vi "Stack_Sequence.vi"() -> ()   [LabVIEW 2016]
panel:
  out "x+y":dbl
  out "Triangle":dynamicdata(graph)
  out "Sine":dynamicdata(graph)
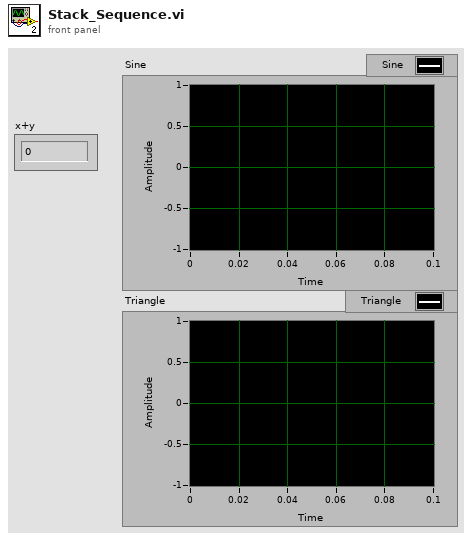
[diagram p1: front panel]
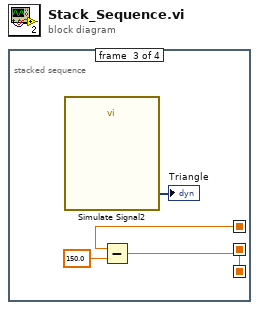
[diagram p0: block diagram]
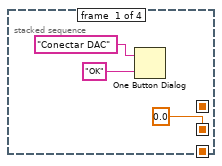
[diagram p2: hidden frame]
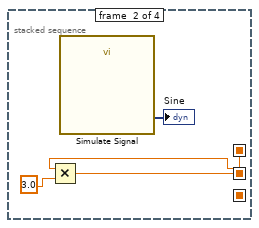
[diagram p3: hidden frame]
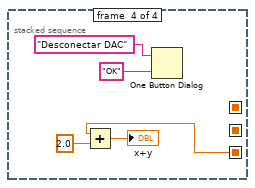
[diagram p4: hidden frame]
diagram:
  n1 = stacked-sequence {
    seq-local: [0.0 _ _ _] -> [_ w5 _ _]
    seq-local: [_ w4 _ _] -> [_ _ w9 _]
    seq-local: [_ _ w8 _] -> [_ _ _ w14]
    frame #0 {
      n2 = One Button Dialog(message="Conectar DAC", button name ("OK")="OK") -> ()  [unwired: 1 out]
    }
    frame #1 {
      n3 = Multiply(x=w5, y=3.0) -> (x*y=w4:dbl)
      n4 = call "Simulate Signal"() -> ("Sine"=→"Sine":dynamicdata)  [unwired: 14 in, 1 out]
    }
    frame #2 {
      n5 = call "Simulate Signal2"() -> ("Triangle"=→"Triangle":dynamicdata)  [unwired: 14 in, 1 out]
      n6 = Subtract(x=w9, y=150.0) -> (x-y=w8:dbl)
    }
    frame #3 {
      n7 = Add(x=w14, y=2.0) -> (x+y=→"x+y":dbl)
      n8 = One Button Dialog(message="Desconectar DAC", button name ("OK")="OK") -> ()  [unwired: 1 out]
    }
  }
